vi "Create and Configure AO.vi"(7 "duration":dbl=1000.0, 8 "error in":errorcluster, 11 "AO channel":string) -> (0 "error out":errorcluster, 3 "AO task":refnum<k21>, 5 "samples":i32)   [LabVIEW 2021, in "audio_frequencyResponseMeasurement.lvlib"]
uses:
  audio_frequencyResponseMeasurement.lvlib
  <resource>/objmgr/daqmx.rc
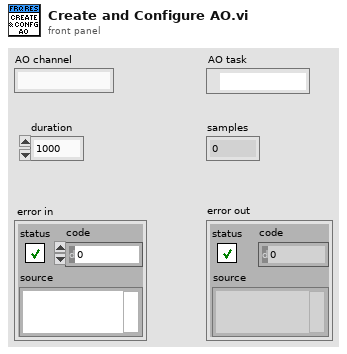
[diagram p1: front panel]
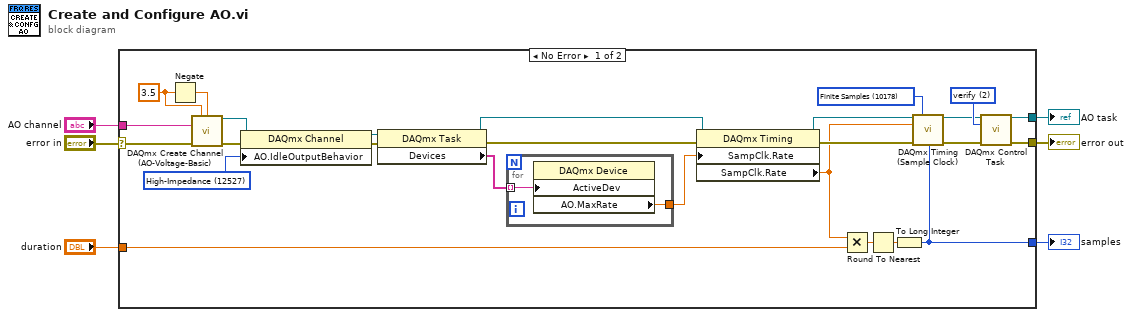
[diagram p0: block diagram]
diagram:
  n1 = case shown="No Error" "error in" {
    selector: "error in" -> [w17 w35]
    tunnel: [w29 _] -> w6
    tunnel: [w28 w35] -> w5
    tunnel: "AO channel" -> [w25 _]
    tunnel: "duration" -> [w14 _]
    tunnel: [w7 _] -> w1
    frame No Error {
      w20 = 12527 items=["Zero Volts"=12526, "High-Impedance"=12527, "Maintain Existing Value"=12528] ("AO.IdleOutputBehavior")
      w26 = 3.5
      w30 = 2 items=["verify"=2, "reserve"=4, "commit"=3, "unreserve"=5, "abort"=6] ("action")
      w31 = 10178 items=["Finite Samples"=10178, "Continuous Samples"=10123, "Hardware Timed Single Point"=12522] ("sample mode")
      n2 = Negate(x=w26) -> (-x=w27:dbl)
      n3 = call <vilib>:"DAQmx Create Channel (AO-Voltage-Basic).vi"("maximum value"=w26, "minimum value"=w27, "physical channels"=w25, "error in"=w17) -> ("task out"=w23:refnum<k21>, "error out"=w24:errorcluster)  [unwired: 10 in]
      n4 = property on="Property Node" class="DAQmx Channel"(reference=w23, error in=w24, "AO.IdleOutputBehavior"=w20) -> (reference out=w22:refnum<k21>, error out=w21:errorcluster)
      n5 = property on="Property Node" class="DAQmx Task"(reference=w22, error in=w21) -> (reference out=w13:refnum<k21>, error out=w11:errorcluster, "Devices"=w32:tag[])
      n6 = for {
        tunnel: w32 -> [w34] mode=indexing
        tunnel: [w33] -> w9
        n7 = property on="Property Node" class="DAQmx Device"("ActiveDev"=w34) -> ("AO.MaxRate"=w33:dbl)  [unwired: 2 in, 2 out]
      }
      n8 = property on="Property Node" class="DAQmx Timing"(reference=w13, error in=w11, "SampClk.Rate"=w9) -> (reference out=w12:refnum<k21>, error out=w10:errorcluster, "SampClk.Rate"=w8:dbl)
      n9 = Multiply(x=w8, y=w14) -> (x*y=w16:dbl)
      n10 = Round To Nearest(number=w16) -> (nearest integer value=w15:dbl)
      n11 = To Long Integer(number=w15) -> (32bit integer=w7:i32)
      n12 = call <vilib>:"DAQmx Timing (Sample Clock).vi"("task/channels in"=w12, "sample mode"=w31, "samples per channel"=w7, "rate"=w8, "error in"=w10) -> ("task out"=w19:refnum<k21>, "error out"=w18:errorcluster)  [unwired: 9 in]
      n13 = call <vilib>:"DAQmx Control Task.vi"("task/channels in"=w19, "action"=w30, "error in"=w18) -> ("task out"=w29:refnum<k21>, "error out"=w28:errorcluster)  [unwired: 11 in]
    }
    frame Error {
    }
  }
  "AO task" <- w6
  "error out" <- w5
  "samples" <- w1
